vi "XY Graph Set Plot Metdata.vi"(8 "error in (no error)":errorcluster, 9 "Plot Metadata":variant, 10 "Plot Index (-1: last)":i32=-1, 11 "XYGraph Ref in":T1) -> (0 "error out":errorcluster, 1 "Plot Name":string, 3 "XY Graph Caption (or Label)":string)   [LabVIEW 2019]
uses:
  XY Graph Refnum.ctl
  XY Graph Add-Ons.lvlib
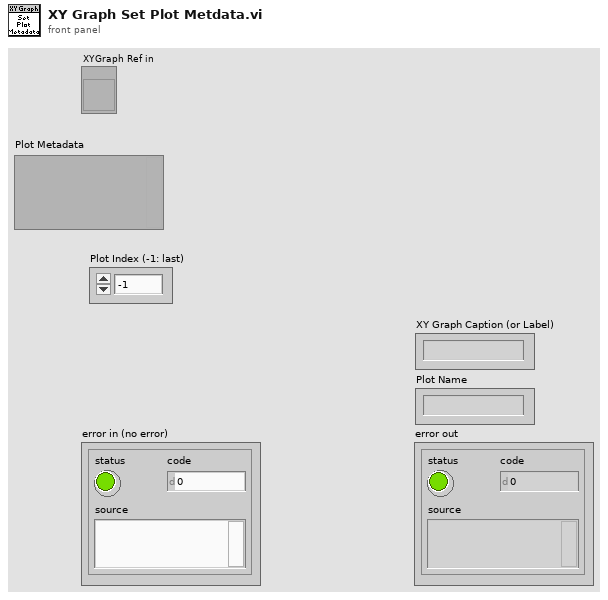
[diagram p1: front panel]
types:
  T1 = typedef "XY Graph Add-Ons.lvlib/XY Graph Refnum.ctl" = refnum<vi>
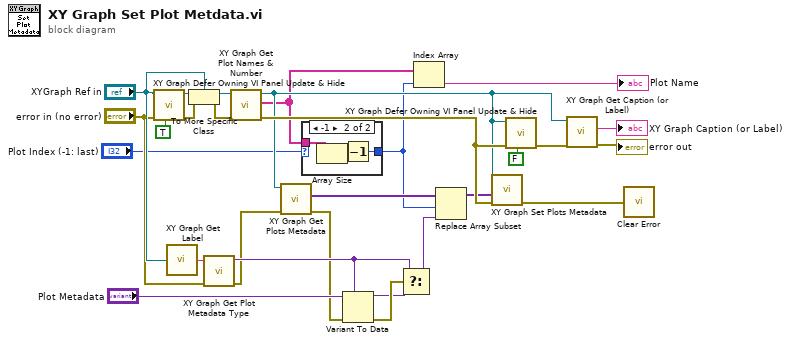
[diagram p0: block diagram]
diagram:
  n1 = call "XY Graph Defer Owning VI Panel Update & Hide.vi"("Defer Owning Panel Update"=TRUE, "error in (no error)"="error in (no error)", "XY Graph Refnum in"="XYGraph Ref in") -> ("error out"=w23:errorcluster, "XY Graph Refnum out"=w26:refnum<vi>)  [unwired: 7 in]
  n2 = call "XY Graph Get Label.vi"("XYGraph"="XYGraph Ref in") -> ("Graph Label"=w15:string)  [unwired: 8 in]
  n3 = To More Specific Class(target class="XYGraph Ref in", reference=w26, error in=w23) -> (specific class reference=w24:T1, error out=w22:errorcluster)
  n4 = call "XY Graph Get Plot Metadata Type.vi"("Error In"="error in (no error)", "Graph Label"=w15) -> ("Error Out"=w8:errorcluster, "Plot Metadata Type"=w10:variant)  [unwired: 7 in, 1 out]
  n5 = call "XY Graph Get Plot Names & Number.vi"("error in (no error)"=w22, "XYGraph in"=w24) -> ("error out"=w28:errorcluster, "Plot Names"=w1:string[], "XYGraph out"=w6:T1)  [unwired: 5 in, 2 out]
  n6 = call "XY Graph Get Plots Metadata.vi"("Error In"=w8, "XYGraph Refnum"=w6) -> ("Error Out"=w7:errorcluster, "Plots Metadata"=w18:variant[])  [unwired: 6 in, 2 out]
  n7 = case shown="-1" "Plot Index (-1: last)" {
    selector: "Plot Index (-1: last)" -> [w29 _]
    tunnel: [w29 w30] -> w2
    tunnel: w1 -> [_ w32]
    frame 0, Default {
    }
    frame -1 {
      n8 = Array Size(array=w32) -> (size(s)=w31:i32)
      n9 = Decrement(x=w31) -> (x-1=w30:i32)
    }
  }
  n10 = Variant To Data(error in=w7, type=w10, Variant="Plot Metadata") -> (data=w9:variant, error out=w11:errorcluster)
  n11 = Select(t=w10, s=w11, f=w9) -> (s? t:f=w5:variant)
  n12 = Index Array(array=w1, index=w2) -> (element=→"Plot Name":string)
  n13 = Replace Array Subset(array=w18, new element=w5, index=w2) -> (w17:variant[])
  n14 = call "XY Graph Set Plots Metadata.vi"("error in (no error)"=w28, "Plots Metadata"=w17, "XY Graph Refnum"=w6) -> ("error out"=w16:errorcluster)  [unwired: 7 in, 1 out]
  n15 = call "XY Graph Defer Owning VI Panel Update & Hide.vi"("Defer Owning Panel Update"=FALSE, "error in (no error)"=w28, "XY Graph Refnum in"=w6) -> ("error out"=w20:errorcluster)  [unwired: 7 in, 1 out]
  n16 = call "XY Graph Get Caption (or Label).vi"("error in (no error)"=w20, "XYGraph in"=w6) -> ("error out"=→"error out":errorcluster, "Caption (or Label) Text"=→"XY Graph Caption (or Label)":string)  [unwired: 7 in, 1 out]
  n17 = call "Clear Error.vi"("Error In"=w16) -> ()  [unwired: 8 in, 1 out]
